vi "Generate Content.vi"(5 "Time Format":string, 7 "Msg Pattern":string, 8 "error in (no error)":errorcluster, 9 "Msg":string, 10 "Caller":string, 11 "Log Level":T1) -> (0 "error out":errorcluster, 2 "Content":string)   [LabVIEW 2020, in "Logging.lvlib"]
uses:
  Logging.lvlib
  Define/Log Level.ctl
  <vilib>/regexp/Match Regular Expression.xnode
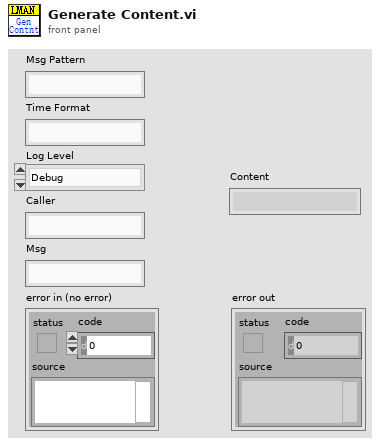
[diagram p1: front panel]
types:
  T1 = typedef "Logging.lvlib/Log Level.ctl" = enum16{"Debug", "Info", "Warn", "Error"}
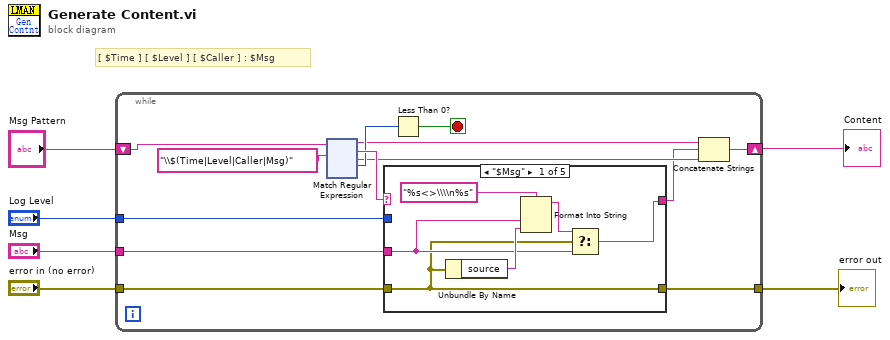
[diagram p0: block diagram]
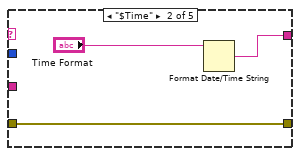
[diagram p2: hidden frame]
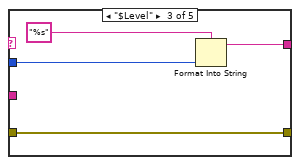
[diagram p3: hidden frame]
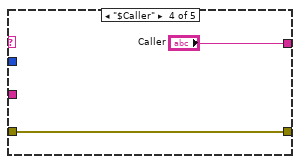
[diagram p4: hidden frame]
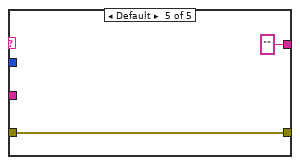
[diagram p5: hidden frame]
diagram:
  # "[ $Time ] [ $Level ] [ $Caller ] : $Msg"
  n1 = while {
    shift-right: [w8] -> w4
    shift-left: "Msg Pattern" -> [w19]
    tunnel: "error in (no error)" -> [w12]
    tunnel: "Log Level" -> [w14]
    tunnel: "Msg" -> [w13]
    tunnel: [w7] -> w1
    stop <- w15 stop-if-true
    n2 = xnode "Match Regular Expression"("input string"=w19, "regular expression"="\\$(Time|Level|Caller|Msg)") -> ("before match"=w11:string, "whole match"=w18:string, "after match"=w10:string, "offset past match"=w16:i32)  [unwired: 4 in, 1 out]
    n3 = case shown="\"$Msg\"" w18 {
      tunnel: w14 -> [_ _ w31 _ _]
      tunnel: w13 -> [w21 _ _ _ _]
      tunnel: w12 -> [w20 w26 w29 w34 w36]
      tunnel: [w25 w27 w30 "Caller" "" ("Caller")] -> w9
      tunnel: [w20 w26 w29 w34 w36] -> w7
      frame "$Msg" {
        n4 = Unbundle By Name(w20) -> ("source"=w22:string)
        n5 = Format Into String(format string="%s<>\\\\n%s", w21, w22) -> (resulting string=w23:string)  [unwired: 2 in, 1 out]
        n6 = Select(t=w23, s=w20, f=w21) -> (s? t:f=w25:string)
      }
      frame "$Time" {
        n7 = Format Date/Time String(time format string (%c)="Time Format") -> (date/time string=w27:string)  [unwired: 2 in]
      }
      frame "$Level" {
        n8 = Format Into String(format string="%s", w31) -> (resulting string=w30:string)  [unwired: 2 in, 1 out]
      }
      frame "$Caller" {
      }
      frame Default {
      }
    }
    n9 = Less Than 0?(x=w16) -> (x < 0?=w15:bool)
    n10 = Concatenate Strings(w11, w9, w10) -> (w8:string)
  }
  "Content" <- w4
  "error out" <- w1
